vi "Voltage - Continuous Output.vi"() -> ()   [LabVIEW 2014]
doc: "本范例演示从计算机内存缓冲区连续重新生成数据的方法。\n\n关于引脚和硬件功能的信息，见设备相关的文档。"
uses:
  <vilib>/Utility/error.llb/DialogType.ctl
  <vilib>/DAQmx/write.llb/DAQmx Write (Analog 1D Wfm NChan NSamp).vi
  <vilib>/DAQmx/create/channels.llb/DAQmx Create Channel (AO-Voltage-Basic).vi
  <vilib>/DAQmx/configure/timing.llb/DAQmx Timing (Sample Clock).vi
  <vilib>/DAQmx/configure/trigger.llb/DAQmx Start Trigger (Digital Edge).vi
  <vilib>/DAQmx/configure/trigger.llb/DAQmx Start Trigger (Analog Edge).vi
  <vilib>/DAQmx/miscellaneous.llb/DAQmx Fill In Error Info.vi
  <resource>/objmgr/daqmx.rc
  <vilib>/measure/NI_MABase.lvlib
panel:
  in  "触发类型":T1(tab)
  in  "Digital Start Trigger Edge":i32(ring)=10280 caption="Edge" items=["Rising"=10280, "Falling"=10171]
  in  "Digital Start Trigger Source":tag="/Dev1/PFI0" caption="Source"
  in  "Digital Pause Trigger Pause When":i32(ring)=10192 caption="Pause When" items=["High"=10192, "Low"=10214]
  in  "Digital Pause Trigger Source":tag="/Dev1/PFI0" caption="Source"
  in  "Analog Start Trigger Level":dbl caption="Level" format="%0.2f"
  in  "Analog Start Trigger Hysteresis":dbl caption="Hysteresis" format="%.2f"
  in  "Analog Start Trigger Slope":i32(ring)=10280 caption="Slope" items=["Rising"=10280, "Falling"=10171]
  in  "Analog Start Trigger Source":string="APFI0" caption="Source"
  in  "Analog Pause Trigger Source":string="APFI0" caption="Source"
  in  "Analog Pause Trigger Pause When":i32(ring)=10093 caption="Pause When" items=["Above Level"=10093, "Below Level"=10107]
  in  "Analog Pause Trigger Level":dbl caption="Level" format="%.2f"
  out "实际采样率":dbl=1000.0 format="%0.2f"
  in  "输出数组":cluster{"波形类型":u16, "幅值":dbl, "频率":dbl}[](array[cluster])=[{"波形类型"=0, "幅值"=0.01, "频率"=10.0}] {"频率" format="%0.2p"; "幅值" format="%0.2p"; "波形类型" items=["正弦波", "三角波", "方波", "锯齿波"]}
  in  "采样数":i32=1000
  in  "停止":bool
  out "波形图":waveform(dbl)[](graph)=[{"t0"=timestamp(0 s since 1904-01-01), "dt"=0.001, "Y"=[]}]
  in  "采样率":dbl=1000.0
  in  "采样时钟源":tag="OnboardClock"
  in  "最大电压":dbl=5.0
  in  "最小碘盐":dbl=-5.0
  in  "物理通道":tag="Dev1/ao0"
  # "波形数组中元素的个数，必须等于任务中通道的个数。"
  # "触发设置"
  # "通道设置"
  # "输出"
  # "定时和缓冲设置"
  # "如需配置并使用开始触发，必须先在上面选择相应的选项卡。有些硬件不支持触发－更多信息见设备的相应文档。"
  # "To enable triggers, select a tab above, and configure the settings.\n\nNot all hardware supports all trigger types. Refer to your device documentation for more information."
  # "This trigger type is not supported in output tasks. \n\nRefer to your device documentation for more information on which triggers are supported."
  # "This trigger type is not supported in output tasks. \n\nRefer to your device documentation for more information on which triggers are supported."
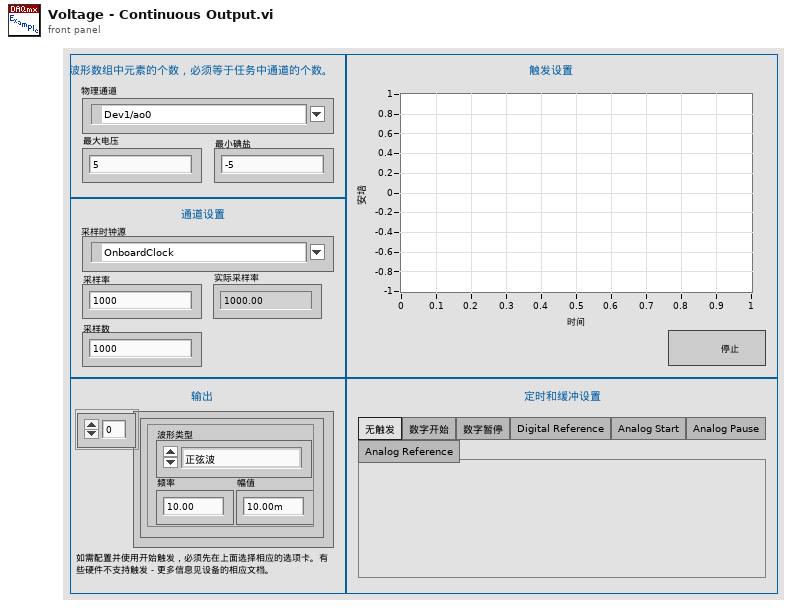
[diagram p1: front panel]
types:
  T1 = enum32{"No Trigger", "Digital Start", "Digital Pause", "Digital Reference", "Analog Start", "Analog Pause", "Analog Reference"}
  T2 = typedef "DialogType.ctl" = u16
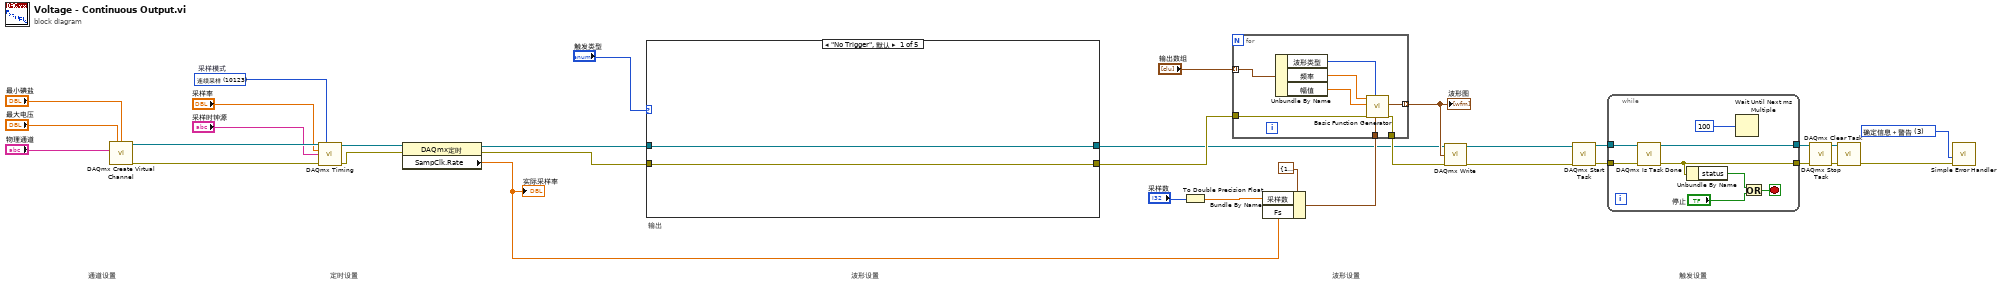
[diagram p0: block diagram]
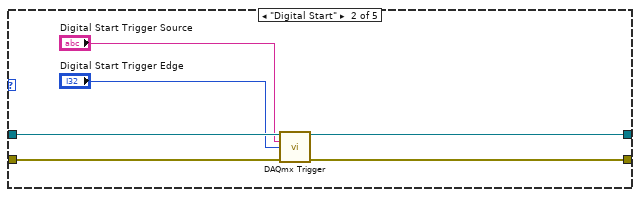
[diagram p2: hidden frame]
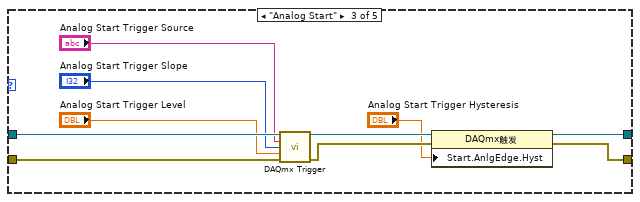
[diagram p3: hidden frame]
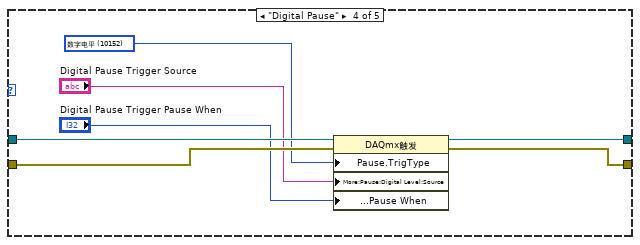
[diagram p4: hidden frame]
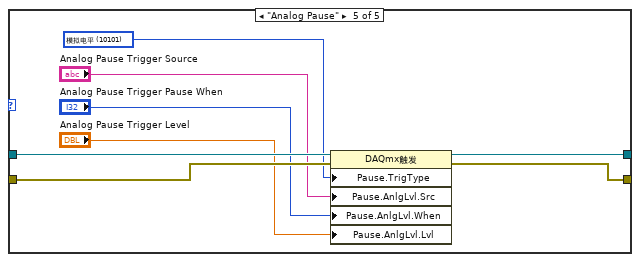
[diagram p5: hidden frame]
diagram:
  w6 = T2 3 items=["无对话框", "确定信息", "继续或停止信息", "确定信息＋警告", "继续/停止＋警告"] ("对话框类型（确定信息：1）")
  w31 = 10123 items=["有限采样"=10178, "连续采样"=10123, "硬件定时单点"=12522]  # 采样模式
  # "波形设置"
  # "输出"
  # "触发设置"
  # "波形设置"
  # "定时设置"
  # "通道设置"
  n1 = call-poly <vilib>:"DAQmx Create Virtual Channel.vi"("maximum value"="最大电压", "minimum value"="最小碘盐", "physical channels"="物理通道") -> ("task out"=w29:refnum<k21>, "error out"=w30:errorcluster)  [unwired: 11 in]
  n2 = call-poly <vilib>:"DAQmx Timing.vi"("task/channels in"=w29, "sample mode"=w31, "rate"="采样率", "source"="采样时钟源", "error in"=w30) -> ("task out"=w33:refnum<k21>, "error out"=w32:errorcluster)  [unwired: 9 in]
  n3 = property class="DAQmx定时"(reference=w33, error in=w32) -> (reference out=w3:refnum<k21>, error out=w4:errorcluster, "SampClk.Rate"=w7:dbl)
  "实际采样率" <- w7
  n4 = case shown="\"No Trigger\", 默认" "触发类型" {
    tunnel: w3 -> [w35 w41 w51 w58 w66]
    tunnel: w4 -> [w34 w40 w50 w55 w63]
    tunnel: [w35 w39 w48 w57 w65] -> w1
    tunnel: [w34 w38 w47 w56 w64] -> w2
    frame "No Trigger", Default {
    }
    frame "Digital Start" {
      n5 = call-poly <vilib>:"DAQmx Trigger.vi"("task/channels in"=w41, "source"="Digital Start Trigger Source", "edge"="Digital Start Trigger Edge", "error in"=w40) -> ("task out"=w39:refnum<k21>, "error out"=w38:errorcluster)  [unwired: 10 in]
    }
    frame "Analog Start" {
      n6 = call-poly <vilib>:"DAQmx Trigger.vi"("task/channels in"=w51, "source"="Analog Start Trigger Source", "slope"="Analog Start Trigger Slope", "level"="Analog Start Trigger Level", "error in"=w50) -> ("task out"=w46:refnum<k21>, "error out"=w45:errorcluster)  [unwired: 9 in]
      n7 = property class="DAQmx触发"(reference=w46, error in=w45, "Start.AnlgEdge.Hyst"="Analog Start Trigger Hysteresis") -> (reference out=w48:refnum<k21>, error out=w47:errorcluster)
    }
    frame "Digital Pause" {
      w54 = 10152 items=["模拟电平"=10101, "模拟窗"=10103, "数字电平"=10152, "数字波形"=10398, "无"=10230] ("Pause.TrigType")
      n8 = property class="DAQmx触发"(reference=w58, error in=w55, "Pause.TrigType"=w54, "More:Pause:Digital Level:Source"="Digital Pause Trigger Source", "More:Pause:Digital Level:Pause When"="Digital Pause Trigger Pause When") -> (reference out=w57:refnum<k21>, error out=w56:errorcluster)
    }
    frame "Analog Pause" {
      w62 = 10101 items=["模拟电平"=10101, "模拟窗"=10103, "数字电平"=10152, "数字波形"=10398, "无"=10230] ("Pause.TrigType")
      n9 = property class="DAQmx触发"(reference=w66, error in=w63, "Pause.TrigType"=w62, "Pause.AnlgLvl.Src"="Analog Pause Trigger Source", "Pause.AnlgLvl.When"="Analog Pause Trigger Pause When", "Pause.AnlgLvl.Lvl"="Analog Pause Trigger Level") -> (reference out=w65:refnum<k21>, error out=w64:errorcluster)
    }
  }
  n10 = To Double Precision Float(number="采样数") -> (double precision float=w14:dbl)
  n11 = Bundle By Name(cluster=cluster{"Fs":dbl, "采样数":dbl} {"Fs"=1000.0, "采样数"=1000.0} ("采样信息"), "采样数"=w14, "Fs"=w7) -> (w19:cluster{"Fs":dbl, "采样数":dbl})
  n12 = for {
    tunnel: w2 -> [w74]
    tunnel: w19 -> [w73]
    tunnel: [w72] -> w16
    tunnel: "输出数组" -> [w71] mode=indexing
    tunnel: [w67] -> w15 mode=indexing
    n13 = Unbundle By Name(w71) -> ("波形类型"=w70:u16, "频率"=w69:dbl, "幅值"=w68:dbl)
    n14 = call <vilib>:"Basic Function Generator.vi"("sampling info"=w73, "signal type"=w70, "error in (no error)"=w74, "amplitude"=w68, "frequency"=w69) -> ("error out"=w72:errorcluster, "signal out"=w67:waveform(dbl))  [unwired: 4 in, 1 out]
  }
  "波形图" <- w15
  n15 = call-poly <vilib>:"DAQmx Write.vi"("task/channels in"=w1, "data"=w15, "error in"=w16) -> ("task out"=w18:refnum<k21>, "error out"=w17:errorcluster)  [unwired: 10 in, 1 out]
  n16 = call <vilib>:"DAQmx Start Task.vi"("task/channels in"=w18, "error in"=w17) -> ("task out"=w28:refnum<k21>, "error out"=w27:errorcluster)  [unwired: 12 in]
  n17 = while {
    tunnel: w28 -> [w82]
    tunnel: w27 -> [w81]
    tunnel: [w78] -> w8
    tunnel: [w79] -> w9
    stop <- w80 stop-if-true
    n18 = call <vilib>:"DAQmx Is Task Done.vi"("task/channels in"=w82, "error in"=w81) -> ("task out"=w79:refnum<k21>, "error out"=w78:errorcluster)  [unwired: 11 in, 1 out]
    n19 = Unbundle By Name(w78) -> ("status"=w77:bool)
    n20 = Wait Until Next ms Multiple(millisecond multiple=u32 100 ("毫秒倍数")) -> ()  [unwired: 1 out]
    n21 = Or(x=w77, y="停止") -> (x .or. y?=w80:bool)
  }
  n22 = call <vilib>:"DAQmx Stop Task.vi"("task/channels in"=w9, "error in"=w8) -> ("task out"=w11:refnum<k21>, "error out"=w10:errorcluster)  [unwired: 12 in]
  n23 = call <vilib>:"DAQmx Clear Task.vi"("task in"=w11, "error in"=w10) -> ("error out"=w26:errorcluster)  [unwired: 13 in]
  n24 = call <vilib>:"Simple Error Handler.vi"("type of dialog (OK msg:1)"=w6, "error in (no error)"=w26) -> ()  [unwired: 3 in, 5 out]
